vi "rszvl_core_global.vi"() -> ()   [LabVIEW 2014] (continued)
\nNote:\n\n(1) Only Upper Limit is available\n\n(7) CATV Digital TV Quadrature Error Limit Result:\nThis attribute performs a limit check for the quadrature error in the Modulation Errors measurement.\n\n(8) CATV Digital TV Symbol Rate Offset Limit Result:\nThis attribute performs a limit check for the symbol rate offset in the Overview measurement.", "Flags"={"OPC Wait"=FALSE, "Dont check status"=FALSE, "*WAI"=FALSE}, "Check Status Callback"=""}, {"Level"=3, "Descriptive Name"="CATV Digital TV Carrier Frequency Offset Limit Result", "Class Only"=FALSE, "Data Type"=0, "Access"=0, "Identifier"="RSZVL_ATTR_CATV_DTV_CARR_LIM_FREQ_OFFSET_RESULT", "Range Table"="rszvl_rngCatvResults", "Command"="CALC:DTV:LIM:RES:CFOF:{ModifLowUpp}?", "Read Callback"="", "Write Callback"="", "Range Callback"="", "Check Callback"="", "Rngtable Callback"="", "Coerce Callback"="", "User Callback"="", "Supported Models"="", "Instrument Options"="", "Repeated Capabilities"="", "Restricted Repeated Capabilities"="", "Help"="This attribute performs a limit check for the carrier frequency offset in the Overview measurement.\n\nAvailable Repeated Capabilities:\nModifLowUpp: Low,Upp\r\n\nRemote-control command(s):\nCALCulate:DTV:LIMit:RESult:CFOFfset:<LOWer | UPPer>?", "Flags"={"OPC Wait"=FALSE, "Dont check status"=FALSE, "*WAI"=FALSE}, "Check Status Callback"=""}, {"Level"=3, "Descriptive Name"="CATV Digital TV Channel Power Limit Result", "Class Only"=FALSE, "Data Type"=0, "Access"=0, "Identifier"="RSZVL_ATTR_CATV_DTV_LIM_CHANNEL_POWER_RESULT", "Range Table"="rszvl_rngCatvResults", "Command"="CALC:DTV:LIM:RES:CHP?", "Read Callback"="", "Write Callback"="", "Range Callback"="", "Check Callback"="", "Rngtable Callback"="", "Coerce Callback"="", "User Callback"="", "Supported Models"="", "Instrument Options"="", "Repeated Capabilities"="", "Restricted Repeated Capabilities"="", "Help"="This attribute queries the result of the Channel Power measurement. Upper and lower limit check can not be handled separately.\n\nAvailable Repeated Capabilities:\nNone\n\nRemote-control command(s):\nCALCulate:DTV:LIMit:RESult:CHPower?", "Flags"={"OPC Wait"=FALSE, "Dont check status"=FALSE, "*WAI"=FALSE}, "Check Status Callback"=""}, {"Level"=3, "Descriptive Name"="CATV Digital TV Carrier Suppression Limit Result", "Class Only"=FALSE, "Data Type"=0, "Access"=0, "Identifier"="RSZVL_ATTR_CATV_DTV_CARR_LIM_CARR_SUPP_RESULT", "Range Table"="rszvl_rngCatvResults", "Command"="CALC:DTV:LIM:RES:CSUP:{ModifLowUpp}?", "Read Callback"="", "Write Callback"="", "Range Callback"="", "Check Callback"="", "Rngtable Callback"="", "Coerce Callback"="", "User Callback"="", "Supported Models"="", "Instrument Options"="", "Repeated Capabilities"="", "Restricted Repeated Capabilities"="", "Help"="This attribute performs a limit check for the lower limit of the carrier suppression in the Modulation Errors measurement.\n\nAvailable Repeated Capabilities:\nModifLowUpp: Low,Upp\r\n\nRemote-control command(s):\nCALCulate:DTV:LIMit:RESult:CSUPpression<[:LOWer] | UPPer>?", "Flags"={"OPC Wait"=FALSE, "Dont check status"=FALSE, "*WAI"=FALSE}, "Check Status Callback"=""}, {"Level"=3, "Descriptive Name"="CATV Digital TV Error Limit Result", "Class Only"=FALSE, "Data Type"=0, "Access"=0, "Identifier"="RSZVL_ATTR_CATV_DTV_LIM_ERROR_RESULT", "Range Table"="rszvl_rngCatvResults", "Command"="CALC:DTV:LIM:RES:{DtvErrorMeas}:{ModifLowUpp}?", "Read Callback"="", "Write Callback"="", "Range Callback"="", "Check Callback"="", "Rngtable Callback"="", "Coerce Callback"="", "User Callback"="", "Supported Models"="", "Instrument Options"="", "Repeated Capabilities"="", "Restricted Repeated Capabilities"="", "Help"="This attribute performs an limit check for the Overview/Modulation Errors measurement.\n\nAvailable Repeated Capabilities:\nDtvErrorMeas: EVMPeak,EVMRms,MERPeak,MERRms\r\nModifLowUpp: Low,Upp\r\n\nRemote-control command(s):\nCALCulate:DTV:LIMit:RESult:<EVMPeak | EVMRms | MERPeak | MERRms>:<LOWer | UPPer>?", "Flags"={"OPC Wait"=FALSE, "Dont check status"=FALSE, "*WAI"=FALSE}, "Check Status Callback"=""}, {"Level"=3, "Descriptive Name"="CATV Digital TV IQ Imbalance Limit Result", "Class Only"=FALSE, "Data Type"=0, "Access"=0, "Identifier"="RSZVL_ATTR_CATV_DTV_LIM_IMB_RESULT", "Range Table"="rszvl_rngCatvResults", "Command"="CALC:DTV:LIM:RES:IMB:{ModifLowUpp}?", "Read Callback"="", "Write Callback"="", "Range Callback"="", "Check Callback"="", "Rngtable Callback"="", "Coerce Callback"="", "User Callback"="", "Supported Models"="", "Instrument Options"="", "Repeated Capabilities"="", "Restricted Repeated Capabilities"="", "Help"="This attribute performs a limit check for the I/Q amplitude imbalance value in the Modulation Errors measurement.\n\nAvailable Repeated Capabilities:\nModifLowUpp: Low,Upp\r\n\nRemote-control command(s):\nCALCulate:DTV:LIMit:RESult:IMBalance:<LOWer | UPPer>?", "Flags"={"OPC Wait"=FALSE, "Dont check status"=FALSE, "*WAI"=FALSE}, "Check Status Callback"=""}, {"Level"=3, "Descriptive Name"="CATV Digital TV Phase Jitter Limit Result", "Class Only"=FALSE, "Data Type"=0, "Access"=0, "Identifier"="RSZVL_ATTR_CATV_DTV_LIM_PJIT_RESULT", "Range Table"="rszvl_rngCatvResults", "Command"="CALC:DTV:LIM:RES:PJIT:{ModifLowUpp}?", "Read Callback"="", "Write Callback"="", "Range Callback"="", "Check Callback"="", "Rngtable Callback"="", "Coerce Callback"="", "User Callback"="", "Supported Models"="", "Instrument Options"="", "Repeated Capabilities"="", "Restricted Repeated Capabilities"="", "Help"="This attribute performs an limit check for the phase jitter in the Modulation Errors measurement.\n\nNote:\n\n(1) Only Upper Limit is available\n\nAvailable Repeated Capabilities:\nModifLowUpp: Low,Upp\r\n\nRemote-control command(s):\nCALCulate:DTV:LIMit:RESult:PJITter[:UPPer]?", "Flags"={"OPC Wait"=FALSE, "Dont check status"=FALSE, "*WAI"=FALSE}, "Check Status Callback"=""}, {"Level"=3, "Descriptive Name"="CATV Digital TV Quadrature Error Limit Result", "Class Only"=FALSE, "Data Type"=0, "Access"=0, "Identifier"="RSZVL_ATTR_CATV_DTV_LIM_QERR_RESULT", "Range Table"="rszvl_rngCatvResults", "Command"="CALC:DTV:LIM:RES:QERR:{ModifLowUpp}?", "Read Callback"="", "Write Callback"="", "Range Callback"="", "Check Callback"="", "Rngtable Callback"="", "Coerce Callback"="", "User Callback"="", "Supported Models"="", "Instrument Options"="", "Repeated Capabilities"="", "Restricted Repeated Capabilities"="", "Help"="This attribute performs a limit check for the quadrature error in the Modulation Errors measurement.\n\nAvailable Repeated Capabilities:\nModifLowUpp: Low,Upp\r\n\nRemote-control command(s):\nCALCulate:DTV:LIMit:RESult:QERRor:<LOWer | UPPer>?", "Flags"={"OPC Wait"=FALSE, "Dont check status"=FALSE, "*WAI"=FALSE}, "Check Status Callback"=""}, {"Level"=3, "Descriptive Name"="CATV Digital TV Symbol Rate Offset Limit Result", "Class Only"=FALSE, "Data Type"=0, "Access"=0, "Identifier"="RSZVL_ATTR_CATV_DTV_LIM_SYMB_RATE_OFFSET_RESULT", "Range Table"="rszvl_rngCatvResults", "Command"="CALC:DTV:LIM:RES:SROF:{ModifLowUpp}?", "Read Callback"="", "Write Callback"="", "Range Callback"="", "Check Callback"="", "Rngtable Callback"="", "Coerce Callback"="", "User Callback"="", "Supported Models"="", "Instrument Options"="", "Repeated Capabilities"="", "Restricted Repeated Capabilities"="", "Help"="This attribute performs a limit check for the symbol rate offset in the Overview measurement.\n\nAvailable Repeated Capabilities:\nModifLowUpp: Low,Upp\r\n\nRemote-control command(s):\nCALCulate:DTV:LIMit:RESult:SROFfset:<LOWer | UPPer>?", "Flags"={"OPC Wait"=FALSE, "Dont check status"=FALSE, "*WAI"=FALSE}, "Check Status Callback"=""}, {"Level"=2, "Descriptive Name"="DTV Results", "Class Only"=TRUE, "Data Type"=0, "Access"=0, "Identifier"="", "Range Table"="", "Command"="", "Read Callback"="", "Write Callback"="", "Range Callback"="", "Check Callback"="", "Rngtable Callback"="", "Coerce Callback"="", "User Callback"="", "Supported Models"="", "Instrument Options"="", "Repeated Capabilities"="", "Restricted Repeated Capabilities"="", "Help"="Attributes that return DTV measurement results.\n\n(1) CATV Get Digital TV Spectrum Shoulder Attenuation:\nThis attribute reads the shoulder attenuation value for the digital TV measurements.\n\n(2) CATV Get Digital TV Error:\nThis attribute reads the error rate value for the digital TV measurements.\n\n(3) CATV Get Digital TV Overview Carrier Frequency Offset:\nThis attribute reads the carrier frequency offset value for the digital TV measurements.\n\n(4) CATV Get Digital TV Overview Symbol Rate Offset:\nThis attribute reads the symbol rate offset value for the digital TV measurements.\n\n(5) CATV Get Digital TV Amplitude Imbalance:\nThis attribute reads the amplitude imbalance value for the digital TV measurements.\n\n(6) CATV Get Digital TV Quadrature Error:\nThis attribute reads the quadrature error value for the digital TV measurements.\n\n(7) CATV Get Digital TV Carrier Suppression:\nThis attribute reads the carrier suppression value for the digital TV measurements.\n\n(8) CATV Get Digital TV Phase Jitter:\nThis attribute reads the phase jitter value for the digital TV measurements.\n\n(9) CATV Get Digital TV Channel Power Result:\nThis attribute returns the result value of Channel Power measurement.", "Flags"={"OPC Wait"=FALSE, "Dont check status"=FALSE, "*WAI"=FALSE}, "Check Status Callback"=""}, {"Level"=3, "Descriptive Name"="CATV Get Digital TV Spectrum Shoulder Attenuation", "Class Only"=FALSE, "Data Type"=1, "Access"=0, "Identifier"="RSZVL_ATTR_CATV_DTV_SPEC", "Range Table"="", "Command"="CALC:DTV:RES? {DtvShoulderAtt}", "Read Callback"="", "Write Callback"="", "Range Callback"="", "Check Callback"="", "Rngtable Callback"="", "Coerce Callback"="", "User Callback"="", "Supported Models"="", "Instrument Options"="", "Repeated Capabilities"="", "Restricted Repeated Capabilities"="", "Help"="This attribute reads the shoulder attenuation value for the digital TV measurements.\n\nAvailable Repeated Capabilities:\nDtvShoulderAtt: SAttLow,SAttUpp\r\n\nRemote-control command(s):\nCALCulate<1|2>:DTV:RESult? SALower | SAUPper", "Flags"={"OPC Wait"=FALSE, "Dont check status"=FALSE, "*WAI"=FALSE}, "Check Status Callback"=""}, {"Level"=3, "Descriptive Name"="CATV Get Digital TV Error", "Class Only"=FALSE, "Data Type"=1, "Access"=0, "Identifier"="RSZVL_ATTR_CATV_DTV_ERROR", "Range Table"="", "Command"="CALC:DTV:RES? {DtvErrorMeas}", "Read Callback"="", "Write Callback"="", "Range Callback"="", "Check Callback"="", "Rngtable Callback"="", "Coerce Callback"="", "User Callback"="", "Supported Models"="", "Instrument Options"="", "Repeated Capabilities"="", "Restricted Repeated Capabilities"="", "Help"="This attribute reads the error rate value for the digital TV measurements.\n\nAvailable Repeated Capabilities:\nDtvErrorMeas: EVMPeak,EVMRms,MERPeak,MERRms\r\n\nRemote-control command(s):\nCALCulate<1|2>:DTV:RESult? EVMPeak | EVMRms | MERPeak | MERRms", "Flags"={"OPC Wait"=FALSE, "Dont check status"=FALSE, "*WAI"=FALSE}, "Check Status Callback"=""}, {"Level"=3, "Descriptive Name"="CATV Get Digital TV Overview Carrier Frequency Offset", "Class Only"=FALSE, "Data Type"=1, "Access"=0, "Identifier"="RSZVL_ATTR_CATV_DTV_OVER_CARR_FREQ_OFFSET", "Range Table"="", "Command"="CALC:DTV:RES? CFOF", "Read Callback"="", "Write Callback"="", "Range Callback"="", "Check Callback"="", "Rngtable Callback"="", "Coerce Callback"="", "User Callback"="", "Supported Models"="", "Instrument Options"="", "Repeated Capabilities"="", "Restricted Repeated Capabilities"="", "Help"="This attribute reads the carrier frequency offset value for the digital TV measurements.\n\nAvailable Repeated Capabilities:\nNone\n\nRemote-control command(s):\nCALCulate<1|2>:DTV:RESult? CFOFfset", "Flags"={"OPC Wait"=FALSE, "Dont check status"=FALSE, "*WAI"=FALSE}, "Check Status Callback"=""}, {"Level"=3, "Descriptive Name"="CATV Get Digital TV Overview Symbol Rate Offset", "Class Only"=FALSE, "Data Type"=1, "Access"=0, "Identifier"="RSZVL_ATTR_CATV_DTV_OVER_SRATE_OFFSET", "Range Table"="", "Command"="CALC:DTV:RES? SROF", "Read Callback"="", "Write Callback"="", "Range Callback"="", "Check Callback"="", "Rngtable Callback"="", "Coerce Callback"="", "User Callback"="", "Supported Models"="", "Instrument Options"="", "Repeated Capabilities"="", "Restricted Repeated Capabilities"="", "Help"="This attribute reads the symbol rate offset value for the digital TV measurements.\n\nAvailable Repeated Capabilities:\nNone\n\nRemote-control command(s):\nCALCulate<1|2>:DTV:RESult? SROFfset", "Flags"={"OPC Wait"=FALSE, "Dont check status"=FALSE, "*WAI"=FALSE}, "Check Status Callback"=""}, {"Level"=3, "Descriptive Name"="CATV Get Digital TV Amplitude Imbalance", "Class Only"=FALSE, "Data Type"=1, "Access"=0, "Identifier"="RSZVL_ATTR_CATV_DTV_MERR_IMB", "Range Table"="", "Command"="CALC:DTV:RES? IMB", "Read Callback"="", "Write Callback"="", "Range Callback"="", "Check Callback"="", "Rngtable Callback"="", "Coerce Callback"="", "User Callback"="", "Supported Models"="", "Instrument Options"="", "Repeated Capabilities"="", "Restricted Repeated Capabilities"="", "Help"="This attribute reads the amplitude imbalance value for the digital TV measurements.\n\nAvailable Repeated Capabilities:\nNone\n\nRemote-control command(s):\nCALCulate<1|2>:DTV:RESult? IMBalance", "Flags"={"OPC Wait"=FALSE, "Dont check status"=FALSE, "*WAI"=FALSE}, "Check Status Callback"=""}, {"Level"=3, "Descriptive Name"="CATV Get Digital TV Quadrature Error", "Class Only"=FALSE, "Data Type"=1, "Access"=0, "Identifier"="RSZVL_ATTR_CATV_DTV_MERR_QERR", "Range Table"="", "Command"="CALC:DTV:RES? QERR", "Read Callback"="", "Write Callback"="", "Range Callback"="", "Check Callback"="", "Rngtable Callback"="", "Coerce Callback"="", "User Callback"="", "Supported Models"="", "Instrument Options"="", "Repeated Capabilities"="", "Restricted Repeated Capabilities"="", "Help"="This attribute reads the quadrature error value for the digital TV measurements.\n\nAvailable Repeated Capabilities:\nNone\n\nRemote-control command(s):\nCALCulate<1|2>:DTV:RESult? QERRor", "Flags"={"OPC Wait"=FALSE, "Dont check status"=FALSE, "*WAI"=FALSE}, "Check Status Callback"=""}, {"Level"=3, "Descriptive Name"="CATV Get Digital TV Carrier Suppression", "Class Only"=FALSE, "Data Type"=1, "Access"=0, "Identifier"="RSZVL_ATTR_CATV_DTV_MERR_CSUP", "Range Table"="", "Command"="CALC:DTV:RES? CSUP", "Read Callback"="", "Write Callback"="", "Range Callback"="", "Check Callback"="", "Rngtable Callback"="", "Coerce Callback"="", "User Callback"="", "Supported Models"="", "Instrument Options"="", "Repeated Capabilities"="", "Restricted Repeated Capabilities"="", "Help"="This attribute reads the carrier suppression value for the digital TV measurements.\n\nAvailable Repeated Capabilities:\nNone\n\nRemote-control command(s):\nCALCulate<1|2>:DTV:RESult? CSUPpression", "Flags"={"OPC Wait"=FALSE, "Dont check status"=FALSE, "*WAI"=FALSE}, "Check Status Callback"=""}, {"Level"=3, "Descriptive Name"="CATV Get Digital TV Phase Jitter", "Class Only"=FALSE, "Data Type"=1, "Access"=0, "Identifier"="RSZVL_ATTR_CATV_DTV_MERR_PJIT", "Range Table"="", "Command"="CALC:DTV:RES? PJIT", "Read Callback"="", "Write Callback"="", "Range Callback"="", "Check Callback"="", "Rngtable Callback"="", "Coerce Callback"="", "User Callback"="", "Supported Models"="", "Instrument Options"="", "Repeated Capabilities"="", "Restricted Repeated Capabilities"="", "Help"="This attribute reads the phase jitter value for the digital TV measurements.\n\nAvailable Repeated Capabilities:\nNone\n\nRemote-control command(s):\nCALCulate<1|2>:DTV:RESult? PJITter", "Flags"={"OPC Wait"=FALSE, "Dont check status"=FALSE, "*WAI"=FALSE}, "Check Status Callback"=""}, {"Level"=3, "Descriptive Name"="CATV Get Digital TV Channel Power Result", "Class Only"=FALSE, "Data Type"=1, "Access"=0, "Identifier"="RSZVL_ATTR_CATV_DTV_CHANNEL_POWER_RESULT", "Range Table"="", "Command"="CALC:MARK:FUNC:POW:RES? CPOW", "Read Callback"="", "Write Callback"="", "Range Callback"="", "Check Callback"="", "Rngtable Callback"="", "Coerce Callback"="", "User Callback"="", "Supported Models"="", "Instrument Options"="", "Repeated Capabilities"="", "Restricted Repeated Capabilities"="", "Help"="This attribute returns the result value of Channel Power measurement.\n\nAvailable Repeated Capabilities:\nNone\n\nRemote-control command(s):\nCALCulate<1|2>:MARKer:FUNCtion:POWer:RESult? CPOWer", "Flags"={"OPC Wait"=FALSE, "Dont check status"=FALSE, "*WAI"=FALSE}, "Check Status Callback"=""}, {"Level"=2, "Descriptive Name"="TV Analyzer Settings", "Class Only"=TRUE, "Data Type"=0, "Access"=0, "Identifier"="", "Range Table"="", "Command"="", "Read Callback"="", "Write Callback"="", "Range Callback"="", "Check Callback"="", "Rngtable Callback"="", "Coerce Callback"="", "User Callback"="", "Supported Models"="", "Instrument Options"="", "Repeated Capabilities"="", "Restricted Repeated Capabilities"="", "Help"="Attributes that configure TV Analyzer Settings.\n\n(1) CATV TV Analyzer Measurement:\nThis attribute defines the TV Analyzer measurement type.\n\n(2) CATV TV Analyzer Channel:\nThis attribute activates the selected channel table.\n\n(3) CATV TV Analyzer Activate Modulation Standard for Tilt:\nThis attribute activates a modulation standard for the Tilt measurement.\n\n(4) CATV TV Analyzer Deactivate Modulation Standard for Tilt:\nThis attribute deactivates a modulation standard for the Tilt measurement.", "Flags"={"OPC Wait"=FALSE, "Dont check status"=FALSE, "*WAI"=FALSE}, "Check Status Callback"=""}, {"Level"=3, "Descriptive Name"="CATV TV Analyzer Measurement", "Class Only"=FALSE, "Data Type"=0, "Access"=2, "Identifier"="RSZVL_ATTR_CATV_TV_MEAS", "Range Table"="rszvl_rngCatvTvMeas", "Command"="CONF:TV:MEAS", "Read Callback"="", "Write Callback"="", "Range Callback"="", "Check Callback"="", "Rngtable Callback"="", "Coerce Callback"="", "User Callback"="", "Supported Models"="", "Instrument Options"="", "Repeated Capabilities"="", "Restricted Repeated Capabilities"="", "Help"="This attribute defines the TV Analyzer measurement type.\n\nAvailable Repeated Capabilities:\nNone\n\nRemote-control command(s):\nCONFigure:TV:MEASurement TILT", "Flags"={"OPC Wait"=FALSE, "Dont check status"=FALSE, "*WAI"=FALSE}, "Check Status Callback"=""}, {"Level"=3, "Descriptive Name"="CATV TV Analyzer Channel", "Class Only"=FALSE, "Data Type"=2, "Access"=2, "Identifier"="RSZVL_ATTR_CATV_TV_CHANNEL", "Range Table"="", "Command"="CONF:TV:CTAB:SEL", "Read Callback"="", "Write Callback"="rszvl_quotedString_WriteCallback.vi", "Range Callback"="", "Check Callback"="", "Rngtable Callback"="", "Coerce Callback"="", "User Callback"="", "Supported Models"="", "Instrument Options"="", "Repeated Capabilities"="", "Restricted Repeated Capabilities"="", "Help"="This attribute activates the selected channel table.\n\nAvailable Repeated Capabilities:\nNone\n\nRemote-control command(s):\nCONFigure:TV:CTABle:SELect", "Flags"={"OPC Wait"=FALSE, "Dont check status"=FALSE, "*WAI"=FALSE}, "Check Status Callback"=""}, {"Level"=3, "Descriptive Name"="CATV TV Analyzer Activate Modulation Standard for Tilt", "Class Only"=FALSE, "Data Type"=2, "Access"=1, "Identifier"="RSZVL_ATTR_CATV_TV_MOD_STANDARD_TILT_ACTIVATE", "Range Table"="", "Command"="TV:TILT:MST:CEN", "Read Callback"="", "Write Callback"="rszvl_quotedString_WriteCallback.vi", "Range Callback"="", "Check Callback"="", "Rngtable Callback"="", "Coerce Callback"="", "User Callback"="", "Supported Models"="", "Instrument Options"="", "Repeated Capabilities"="", "Restricted Repeated Capabilities"="", "Help"="This attribute activates a modulation standard for the Tilt measurement.\n\nAvailable Repeated Capabilities:\nNone\n\nRemote-control command(s):\n[SENSe<1|2>:]TV:TILT:MSTandard:CENable", "Flags"={"OPC Wait"=FALSE, "Dont check status"=FALSE, "*WAI"=FALSE}, "Check Status Callback"=""}, {"Level"=3, "Descriptive Name"="CATV TV Analyzer Deactivate Modulation Standard for Tilt", "Class Only"=FALSE, "Data Type"=2, "Access"=1, "Identifier"="RSZVL_ATTR_CATV_TV_MOD_STANDARD_TILT_DEACTIVATE", "Range Table"="", "Command"="TV:TILT:MST:CDIS", "Read Callback"="", "Write Callback"="rszvl_quotedString_WriteCallback.vi", "Range Callback"="", "Check Callback"="", "Rngtable Callback"="", "Coerce Callback"="", "User Callback"="", "Supported Models"="", "Instrument Options"="", "Repeated Capabilities"="", "Restricted Repeated Capabilities"="", "Help"="This attribute deactivates a modulation standard for the Tilt measurement.\n\nAvailable Repeated Capabilities:\nNone\n\nRemote-control command(s):\n[SENSe<1|2>:]TV:TILT:MSTandard:CDISable", "Flags"={"OPC Wait"=FALSE, "Dont check status"=FALSE, "*WAI"=FALSE}, "Check Status Callback"=""}, {"Level"=1, "Descriptive Name"="K30 - Noise Figure and Gain Measurments", "Class Only"=TRUE, "Data Type"=0, "Access"=0, "Identifier"="", "Range Table"="", "Command"="", "Read Callback"="", "Write Callback"="", "Range Callback"="", "Check Callback"="", "Rngtable Callback"="", "Coerce Callback"="", "User Callback"="", "Supported Models"="", "Instrument Options"="", "Repeated Capabilities"="", "Restricted Repeated Capabilities"="", "Help"="This class implements attributes of option K30 - Noise Figure and Gain Measurments.\n\n(1) Noise Mode:\nThis attribute selects active operation of the R&S FS-K30 option by specifying its name.\n\n(2) Settings (Class):\nAttributes that configure the settings of Noise measurement.\n\n(3) Display (Class):\nAttributes that configure the display parameters.", "Flags"={"OPC Wait"=FALSE, "Dont check status"=FALSE, "*WAI"=FALSE}, "Check Status Callback"=""}, {"Level"=2, "Descriptive Name"="Noise Mode", "Class Only"=FALSE, "Data Type"=4, "Access"=1, "Identifier"="RSZVL_ATTR_NOISE_MODE", "Range Table"="", "Command"="INST:SEL NOIS", "Read Callback"="", "Write Callback"="", "Range Callback"="", "Check Callback"="", "Rngtable Callback"="", "Coerce Callback"="", "User Callback"="", "Supported Models"="", "Instrument Options"="", "Repeated Capabilities"="", "Restricted Repeated Capabilities"="", "Help"="This attribute selects active operation of the R&S FS-K30 option by specifying its name.\n\nAvailable Repeated Capabilities:\nNone\n\nRemote-control command(s):\nINSTrument:SELect NOIS", "Flags"={"OPC Wait"=FALSE, "Dont check status"=FALSE, "*WAI"=FALSE}, "Check Status Callback"=""}, {"Level"=2, "Descriptive Name"="Settings", "Class Only"=TRUE, "Data Type"=0, "Access"=0, "Identifier"="", "Range Table"="", "Command"="", "Read Callback"="", "Write Callback"="", "Range Callback"="", "Check Callback"="", "Rngtable Callback"="", "Coerce Callback"="", "User Callback"="", "Supported Models"="", "Instrument Options"="", "Repeated Capabilities"="", "Restricted Repeated Capabilities"="", "Help"="Attributes that configure the settings of Noise measurement.\n\n(1) Noise Limit:\nThis attribute assigns a limit line to a particular measurement type. Measurement types include noise figure, noise temperature or gain.\n\n(2) Noise Configure Correction:\nThis attribute configures R&S FS-K30 for a second stage correction measurement.\nAfter this attribute has been executed the second stage correction measurement will be the measurement started when the user issues the INITiate command.\n\n(3) Noise Configure Continuous Frequency List:\nThis attribute configures R&S FS-K30 for a continuous frequency list measurement.\nAfter this attribute has been executed a continuous frequency list measurement will be the measurement started when the user issues the INITiate command.\n\n(4) Noise Configure Single Frequency List:\nThis attribute configures R&S FS-K30 for a single frequency list measurement.\nAfter this attribute has been executed a single frequency list measurement will be the measurement started when the user issues the INITiate command.\n\n(5) Noise Configure Single Measurement:\nThis attribute configures R&S FS-K30 for a single frequency measurement. After this attribute has been executed a single frequency measurement will be the measurement started when the user issues the INITiate command.\n\n(6) Noise Input Pre-selector:\nThis attribute switches the preselection on or off.\n\n(7) Noise Input Pre-amplifier:\nThis attribute switches the pre-amplifier on and off. The B23 option is always required. If only the B2 or B25 option is present in addition to B23 then the pre-amplifier of the installed option is controlled. If both the B2 and B25 options are present then the pre-amplifier controlled by this attirubte depends on the setting for the rszvl_ATTR_NOISE_INP_PRES_STAT attirbute. If the rszvl_ATTR_NOISE_INP_PRES_STAT is set to ON then the pre-amplifier for the B2 option is controlled by this function, otherwise the pre-amplifier of the B25 option is controlled.\n\n(8) Noise ERN Mode Selection:\nThe ENR mode selection attribute is used to specify whether a single ENR spot value applies for all measured frequencies or whether an ENR list table is to be used (ENR values specified at specific input frequencies).\n\n(9) Noise ERN Constant Value:\nThe ENR attribute allows the ENR value applicable to the Noise source for all input frequencies to be specified. This value provides a simple mechanism to enter an ENR value that is\napplicable throughout a range of measurement frequencies.\nThis attribute will however not be effective if\nthe remote control command SENS:CORR:ENR:MODE:TABL was previously entered.\n\n(10) Noise ENR Room Temperature:\nThis ENR attribute allows the room temperature of the operating environment to be specified. This value will be taken into account when calculating noise results. Units are Kelvin.\n\n(11) Noise Loss Mode Selection:\nThis attribute is used to identify whether a single input/output loss value applies for all measured frequencies or whether an input/output loss list is to be used. (Loss Input/Output values specified at specific input frequencies).\n\n(12) Noise Loss Constant Value:\nThis attribute allows the loss input/output constant to be set to a value applicable for all input/output frequencies to be measured. This attribute provides a simple mechanism to enter a loss input/output value that is applicable throughout a range of measurement frequencies.\nThis attribute will however not be effective if the attribute RSZVL_ATTR_NOISE_CORR_LOSS_MODE - TABL was previously entered.\n\n(13) Noise Image Rejection:\nThis attribute allows an image rejection value associated with DUT to be entered which will be effective across the complete range of measurement frequencies.\n\n(14) Noise 2nd State Correction:\nThis attribute can be used to control whether the R&S FS-K30 option will factor in the results obtained from second stage correction when performing a noise and gain measurement.\n\n(15) Noise Frequency Step:\nThis attribute can be used to specify the step frequency for a new frequency measurement list that requires computing. This value will form the basis of one of the input criteria for computing a new frequency list.\n\n(16) Noise Fixed Frequency:\nThis attribute is used to specify a single fixed frequency to measure noise and gain continuously. The value specified with this command is only used when a single frequency measurement is initiated.\n\n(17) Noise Configure Local Oscilator:\nThis attribute can be used to specify whether the local oscillator will be used as a fixed frequency source or a variable frequency source.\nThe attribute will not have any immediate effect if a direct frequency list is being used which is set by the attribute RSZVL_ATTR_NOISE_CONF_MODE_DUT - AMPL.\nSee attribute Noise Configure DUT for an explanation on how the measurement lists are created.\n\nNote:\n\n(1) For R&S FSL is avalilable only FIXed value\n\n(18) Noise Fixed Local Oscilator Frequency:\nThis attribute can be used to specify a fixed local oscillator frequency for a new frequency measurement list that requires computing. This value will form the basis of one of the input criteria for computing a new frequency list.\nThe attribute will not have any immediate effect if a direct frequency list is being used (which is set by the RSZVL_ATTR_NOISE_CONF_MODE_DUT - AMPL attribute) or a variable local osciallator frequency has been specified (which is set by the RSZVL_ATTR_NOISE_CONF_SYST_LOSC - VAR attribute).\n\n(19) Noise Fixed Intermediate Frequency:\nThis attribute can be used to specify a fixed intermediate frequency for a new frequency measurement list that requires computing. This value will form the basis of one of the input criteria for computing a new frequency list.\nThe attribute will not have any immediate effect if a direct frequency list is being used (which is set by the RSZVL_ATTR_NOISE_CONF_MODE_DUT - AMPL attribute) or a variable intermediate frequency has been specified (which is set by the RSZVL_ATTR_NOISE_CONF_SYST_LOSC - VAR attribute).\n\n(20) Noise Configure DUT:\nThis attribute allows the type of DUT to be defined. This setting will determine the method that will be used to create the frequency measurement list. This attribute in addition to Noise Configure Local Oscilator will determine how the DUT is tested. Fixed Local Oscillator or fixed Intermediate Frequencies will be taken from the settings supplied by its functions, where appropriate.\nThe following calculation methods will be used.\nUsing a variable Local Oscillator frequency as set by the attribute RSZVL_ATTR_NOISE_CONF_SYST_LOSC - VAR: i.e. the DUT has a fixed IF frequency.\nUsing a fixed Local Oscillator frequency as set by the attribute RSZVL_ATTR_NOISE_CONF_SYST_LOSC -\nFIX: i.e. the DUT has a variable IF frequency.\nThe attribute will not have any immediate effect if the current frequency measurement mode is\nfixed, as is set by the command SENS:FREQ:MODE FIX.\nRF: = All the above settings for frequency list calculation will calculate the RF frequency for each step.\nThe list of RF frequencies generated will be in the following sequence: Start Frequency, Start\nFrequency + Step Frequency, Start Frequency + Step Frequency*2, Stop Frequency.\nIF: = intermediate frequency\nLO: = local oscillator frequency\n\n(21) Noise External Frequency Offset:\nThis attribute defines the frequency offset of the selected generator with reference to the receive frequency.\nThis attribute is only valid in combination with option Ext. Generator Control R&S FSP-B10. \nNote: Select the frequency offset of the generator so that the frequency range of the generator is not exceeded with the following formula\nGenerator_Frequency = [(LO_Frequency + Offset 1) * Numerator / Denominator)] + Offset 2\nif applied to the start and stop frequency of the analyzer.\n\n(22) Noise External Frequency Numerator:\nThis attribute defines the numerator of the factor with which the analyzer frequency is multiplied in order to obtain the transmit frequency of the selected generator.\nThis attribute is only valid in combination with option Ext. Generator Control R&S FSP-B10.\nNote: Select the multiplication factor in a way that the frequency range of the generator is not\nexceeded by the following formula\nGenerator_Frequency = [(LO_Frequency + Offset 1) * Numerator / Denominator)] + Offset 2\nif applied to the start and stop frequency of the analyzer.\n\n(23) Noise External Frequency Denominator:\nThis attribute defines the denominator of the factor with which the analyzer frequency is multiplied in order to obtain the transmit frequency of the selected generator.\nThis attribute is only valid in combination with option Ext. Generator Control R&S FSP-B10.\nNote: Select the multiplication factor in a way that the frequency range of the generator is not\nexceeded by the following formula\nGenerator_Frequency = [(LO_Frequency + Offset 1) * Numerator / Denominator)] + Offset 2\nif applied to the start and stop frequency of the analyzer.\n\n(24) Noise Output Power Level:\nThis attribute sets the output power of the selected generator. This function is only valid in\ncombination with option Ext. Generator Control R&S FSP-B10.\n\n(25) Noise GPIB Address:\nThis attribute changes the IEC/IEEE-bus address of the external signal generator.\nThe attribute is only available with option Ext. Generator Control B10.\n\n(26) Noise Select Generator:\nThis attribute selects the type of external signal generator. \n\n(27) Noise Generator Automatic Control:\nThis attribute is used to specify whether the setup of the external generator is to be automatically controlled by the R&S FS-K30 option (via GPIB) or manually by the user.\n\n(28) Noise Init Before Measurement:\nThis attribute is used to specify whether an initialisation sequence of GPIB commands is sent to an external signal generator prior to performing each measurement. Sending an initialisation sequence before each measurement ensures that the signal generator will be in the correct state to receive control commands during a measurement sequence, however initialising an external signal generator before each measurement adds a time overhead to each measurement.\n\n(29) Noise Configure Range:\nThis attribute allows the maximum gain of the DUT to be specified.\n\n(30) Noise Settling Time:\nThis attribute allows the DUT settling time to be modified. It represents the time to wait for the DUT to settle after a noise source has been turned on or off.\n\n(31) Noise Save Trace To Memory:\nThis attribute saves the current trace results (noise figure, noise temperature and noise gain traces) to trace memory <n>.", "Flags"={"OPC Wait"=FALSE, "Dont check status"=FALSE, "*WAI"=FALSE}, "Check Status Callback"=""}, {"Level"=3, "Descriptive Name"="Noise Limit", "Class Only"=FALSE, "Data Type"=0, "Access"=2, "Identifier"="RSZVL_ATTR_NOISE_CALC_LIM_TRAC", "Range Table"="rszvl_rngNoiseCalcLimLine", "Command"="CALC:LIM{Limit}:TRAC", "Read Callback"="", "Write Callback"="", "Range Callback"="", "Check Callback"="", "Rngtable Callback"="", "Coerce Callback"="", "User Callback"="", "Supported Models"="", "Instrument Options"="", "Repeated Capabilities"="", "Restricted Repeated Capabilities"="", "Help"="This attribute assigns a limit line to a particular measurement type. Measurement types include noise figure, noise temperature or gain.\n\nAvailable Repeated Capabilities:\nLimit: L1,L2,L3,L4,L5,L6,L7,L8\r\n\nRemote-control command(s):\nCALCulate:LIMit<1..6>:TRACe[?] NFIGure | TEFFective | GAIN", "Flags"={"OPC Wait"=FALSE, "Dont check status"=FALSE, "*WAI"=FALSE}, "Check Status Callback"=""}, {"Level"=3, "Descriptive Name"="Noise Configure Correction", "Class Only"=FALSE, "Data Type"=4, "Access"=1, "Identifier"="RSZVL_ATTR_NOISE_CONF_CORR", "Range Table"="", "Command"="CONF:CORR", "Read Callback"="", "Write Callback"="", "Range Callback"="", "Check Callback"="", "Rngtable Callback"="", "Coerce Callback"="", "User Callback"="", "Supported Models"="", "Instrument Options"="", "Repeated Capabilities"="", "Restricted Repeated Capabilities"="", "Help"="This attribute configures R&S FS-K30 for a second stage correction measurement.\nAfter this attribute has been executed the second stage correction measurement will be the measurement started when the user issues the INITiate command.\n\nAvailable Repeated Capabilities:\nNone\n\nRemote-control command(s):\nCONFigure:CORRection", "Flags"={"OPC Wait"=FALSE, "Dont check status"=FALSE, "*WAI"=FALSE}, "Check Status Callback"=""}, {"Level"=3, "Descriptive Name"="Noise Configure Continuous Frequency List", "Class Only"=FALSE, "Data Type"=4, "Access"=1, "Identifier"="RSZVL_ATTR_NOISE_CONF_LIST_CONT", "Range Table"="", "Command"="CONF:LIST:CONT", "Read Callback"="", "Write Callback"="", "Range Callback"="", "Check Callback"="", "Rngtable Callback"="", "Coerce Callback"="", "User Callback"="", "Supported Models"="", "Instrument Options"="", "Repeated Capabilities"="", "Restricted Repeated Capabilities"="", "Help"="This attribute configures R&S FS-K30 for a continuous frequency list measurement.\nAfter this attribute has been executed a continuous frequency list measurement will be the measurement started when the user issues the INITiate command.\n\nAvailable Repeated Capabilities:\nNone\n\nRemote-control command(s):\nCONFigure:LIST:CONTinuous", "Flags"={"OPC Wait"=FALSE, "Dont check status"=FALSE, "*WAI"=FALSE}, "Check Status Callback"=""}, {"Level"=3, "Descriptive Name"="Noise Configure Single Frequency List", "Class Only"=FALSE, "Data Type"=4, "Access"=1, "Identifier"="RSZVL_ATTR_NOISE_CONF_LIST_SING", "Range Table"="", "Command"="CONF:LIST:SING", "Read Callback"="", "Write Callback"="", "Range Callback"="", "Check Callback"="", "Rngtable Callback"="", "Coerce Callback"="", "User Callback"="", "Supported Models"="", "Instrument Options"="", "Repeated Capabilities"="", "Restricted Repeated Capabilities"="", "Help"="This attribute configures R&S FS-K30 for a single frequency list measurement.\nAfter this attribute has been executed a single frequency list measurement will be the measurement started when the user issues the INITiate command.\n\nAvailable Repeated Capabilities:\nNone\n\nRemote-control command(s):\nCONFigure:LIST:SINGle", "Flags"={"OPC Wait"=FALSE, "Dont check status"=FALSE, "*WAI"=FALSE}, "Check Status Callback"=""}, {"Level"=3, "Descriptive Name"="Noise Configure Single Measurement", "Class Only"=FALSE, "Data Type"=4, "Access"=1, "Identifier"="RSZVL_ATTR_NOISE_CONF_SING", "Range Table"="", "Command"="CONF:SING", "Read Callback"="", "Write Callback"="", "Range Callback"="", "Check Callback"="", "Rngtable Callback"="", "Coerce Callback"="", "User Callback"="", "Supported Models"="", "Instrument Options"="", "Repeated Capabilities"="", "Restricted Repeated Capabilities"="", "Help"="This attribute configures R&S FS-K30 for a single frequency measurement. After this attribute has been executed a single frequency measurement will be the measurement started when the user issues the INITiate command.\n\nAvailable Repeated Capabilities:\nNone\n\nRemote-control command(s):\nCONFigure:SINGle", "Flags"={"OPC Wait"=FALSE, "Dont check status"=FALSE, "*WAI"=FALSE}, "Check Status Callback"=""}, {"Level"=3, "Descriptive Name"="Noise Input Pre-amplifier", "Class Only"=FALSE, "Data Type"=3, "Access"=2, "Identifier"="RSZVL_ATTR_NOISE_INP_GAIN_STAT", "Range Table"="", "Command"="INP:GAIN:STAT", "Read Callback"="", "Write Callback"="", "Range Callback"="", "Check Callback"="", "Rngtable Callback"="", "Coerce Callback"="", "User Callback"="", "Supported Models"="", "Instrument Options"="", "Repeated Capabilities"="", "Restricted Repeated Capabilities"="", "Help"="This attribute switches the pre-amplifier on and off. The B23 option is always required. If only the B2 or B25 option is present in addition to B23 then the pre-amplifier of the installed option is controlled. If both the B2 and B25 options are present then the pre-amplifier controlled by this attirubte depends on the setting for the rszvl_ATTR_NOISE_INP_PRES_STAT attirbute. If the rszvl_ATTR_NOISE_INP_PRES_STAT is set to ON then the pre-amplifier for the B2 option is controlled by this function, otherwise the pre-amplifier of the B25 option is controlled.\n\nAvailable Repeated Capabilities:\nNone\n\nRemote-control command(s):\nINPut:GAIN:STATe[?] ON | OFF", "Flags"={"OPC Wait"=FALSE, "Dont check status"=FALSE, "*WAI"=FALSE}, "Check Status Callback"=""}, {"Level"=3, "Descriptive Name"="Noise ERN Mode Selection", "Class Only"=FALSE, "Data Type"=0, "Access"=2, "Identifier"="RSZVL_ATTR_NOISE_CORR_ENR_MODE", "Range Table"="rszvl_rngNoiseERNModeSel", "Command"="SENS:CORR:ENR:MODE", "Read Callback"="", "Write Callback"="", "Range Callback"="", "Check Callback"="", "Rngtable Callback"="", "Coerce Callback"="", "User Callback"="", "Supported Models"="", "Instrument Options"="", "Repeated Capabilities"="", "Restricted Repeated Capabilities"="", "Help"="The ENR mode selection attribute is used to specify whether a single ENR spot value applies for all 
